vi "RDS Serial Frame Read.vi"(8 "error in (no error)":errorcluster, 11 "RDS Serial Frame in":refnum<class "RDS Serial Frame.lvclass">) -> (0 "error out":errorcluster, 1 "Time Stamp":timestamp, 2 "Serial String":string, 3 "RDS Serial Frame out":refnum<class "RDS Serial Frame.lvclass">)   [LabVIEW 2015, in "RDS Serial Handler.lvlib" / "RDS Serial Frame.lvclass"]
uses:
  RDS Serial Frame.lvclass
  RDS Serial Frame.lvclass/RDS Serial Frame.ctl
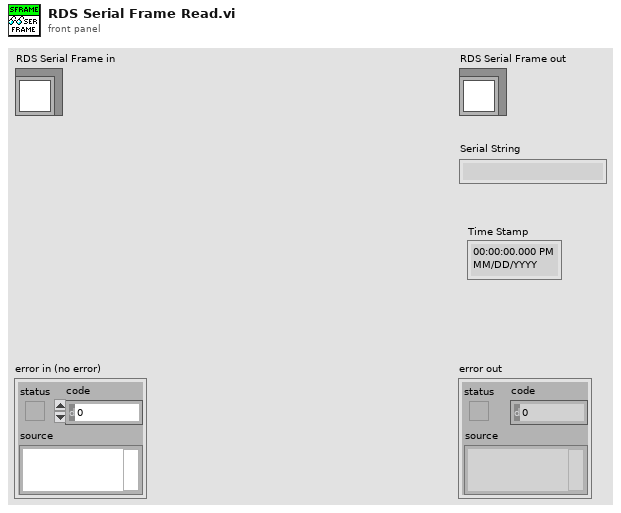
[diagram p1: front panel]
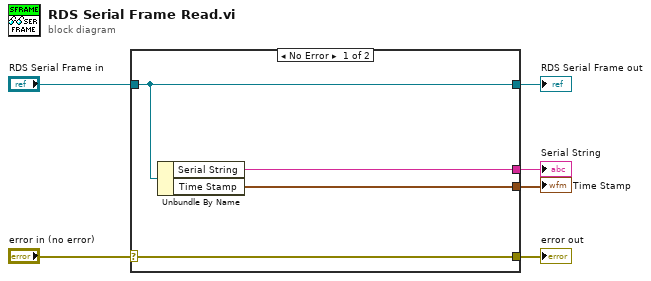
[diagram p0: block diagram]
diagram:
  n1 = case shown="No Error" "error in (no error)" {
    selector: "error in (no error)" -> [w10 w11]
    tunnel: [w10 w11] -> w5
    tunnel: [w9 w12] -> w3
    tunnel: "RDS Serial Frame in" -> [w9 w12]
    tunnel: [w8 _] -> w2
    tunnel: [w7 _] -> w1
    frame No Error {
      n2 = Unbundle By Name(w9) -> ("Serial String"=w8:string, "Time Stamp"=w7:timestamp)
    }
    frame Error {
    }
  }
  "error out" <- w5
  "RDS Serial Frame out" <- w3
  "Serial String" <- w2
  "Time Stamp" <- w1
